vi "Set Value Options.vi"(0 "Control in":refnum<vi>, 5 "type":variant, 7 "populate values":bool, 9 "set default values":bool, 11 "error in (no error)":errorcluster) -> (4 "Control out":refnum<vi>, 15 "error out":errorcluster)   [LabVIEW 2017, in "Variant Control Scripting.lvlib"]
uses:
  Variant Control Scripting.lvlib
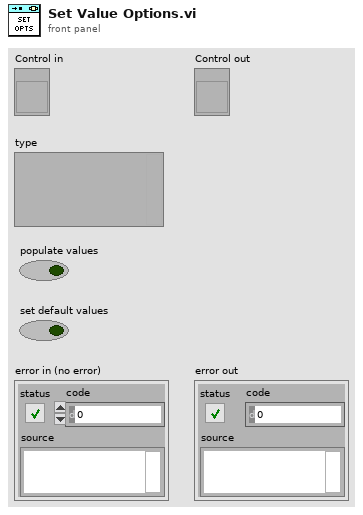
[diagram p1: front panel]
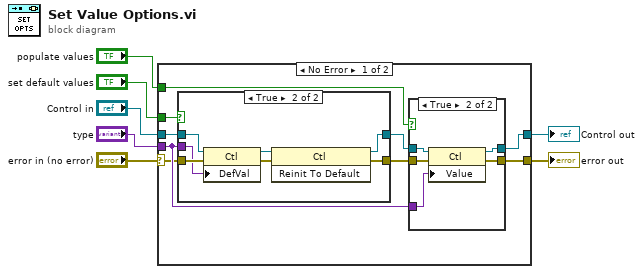
[diagram p0: block diagram]
diagram:
  n1 = case shown="No Error" "error in (no error)" {
    selector: "error in (no error)" -> [w8 w33]
    tunnel: [w16 w34] -> w7
    tunnel: [w15 w33] -> w6
    tunnel: "populate values" -> [w14 _]
    tunnel: "type" -> [w13 _]
    tunnel: "set default values" -> [w10 _]
    tunnel: "Control in" -> [w9 w34]
    frame No Error {
      n2 = case shown="True" w10 {
        tunnel: w8 -> [w24 w32]
        tunnel: [w24 w28] -> w12
        tunnel: [w25 w26] -> w11
        tunnel: w9 -> [w25 w30]
        tunnel: w13 -> [_ w29]
        frame False {
        }
        frame True {
          n3 = property class="Ctl"(reference=w30, error in=w32, "DefVal"=w29) -> (reference out=w27:refnum<vi>, error out=w31:errorcluster)
          n4 = invoke class="Ctl" method="Reinit To Default"(reference=w27, error in=w31) -> (reference out=w26:refnum<vi>, error out=w28:errorcluster)  [unwired: 1 in, 1 out]
        }
      }
      n5 = case shown="True" w14 {
        tunnel: w12 -> [w17 w23]
        tunnel: [w17 w22] -> w15
        tunnel: [w18 w21] -> w16
        tunnel: w11 -> [w18 w20]
        tunnel: w13 -> [_ w19]
        frame False {
        }
        frame True {
          n6 = property class="Ctl"(reference=w20, error in=w23, "Value"=w19) -> (reference out=w21:refnum<vi>, error out=w22:errorcluster)
        }
      }
    }
    frame Error {
    }
  }
  "Control out" <- w7
  "error out" <- w6
